vi "1WIRE_Write_8Bytes.vi"(7 "1-Wire DIO Pin":refnum<k21>="ConnectorA/DIO15", 8 "error in":errorcluster, 10 "Tx data":u64) -> (0 "error out":errorcluster, 2 "Last Written":bool[](array[boolean]))   [LabVIEW 2014]
doc: "This VI is created by Vincent Claes for FPDA-1 more information on http://pwo.fpga.be\n\nvincent.claes@xios.be\nclaesvincent@gmail.com\n\nhttp://www.linkedin.com/in/vincentclaes"
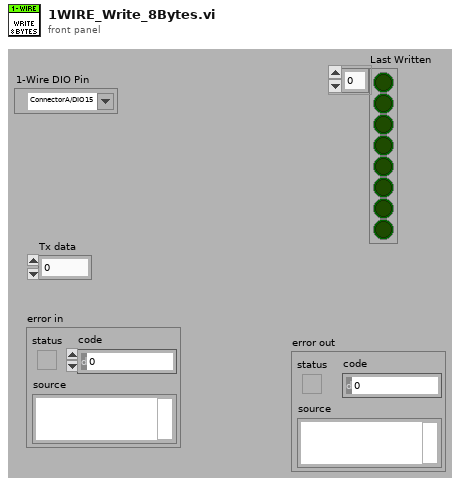
[diagram p1: front panel]
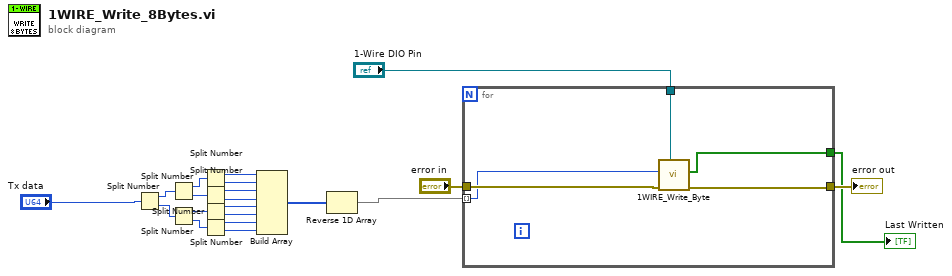
[diagram p0: block diagram]
diagram:
  n1 = Split Number(x="Tx data") -> (hi(x)=w15:u32, lo(x)=w14:u32)
  n2 = Split Number(x=w15) -> (hi(x)=w13:u16, lo(x)=w12:u16)
  n3 = Split Number(x=w14) -> (hi(x)=w11:u16, lo(x)=w10:u16)
  n4 = Split Number(x=w13) -> (hi(x)=w9:u8, lo(x)=w8:u8)
  n5 = Split Number(x=w12) -> (hi(x)=w7:u8, lo(x)=w6:u8)
  n6 = Split Number(x=w11) -> (hi(x)=w5:u8, lo(x)=w4:u8)
  n7 = Split Number(x=w10) -> (hi(x)=w3:u8, lo(x)=w2:u8)
  n8 = Build Array(w9, w8, w7, w6, w5, w4, w3, w2) -> (w1:u8[])
  n9 = Reverse 1D Array(array=w1) -> (reversed array=w17:u8[])
  n10 = for {
    tunnel: [w24] -> w21
    tunnel: "error in" -> [w25]
    tunnel: "1-Wire DIO Pin" -> [w26]
    tunnel: w17 -> [w23] mode=indexing
    tunnel: [w22] -> w16
    n11 = call "1WIRE_Write_Byte.vi"("1-Wire DIO Pin"=w26, "error in"=w25, "Tx data"=w23) -> ("error out"=w24:errorcluster, "Written"=w22:bool[])  [unwired: 7 in]
  }
  "error out" <- w21
  "Last Written" <- w16
